vi "AVTCP-Test Client.vi"() -> ()   [LabVIEW 2016]
panel:
  out "result":i32
  in  "Send":bool
  in  "stop":bool
  in  "Message":string
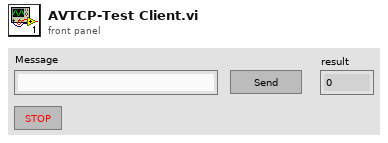
[diagram p1: front panel]
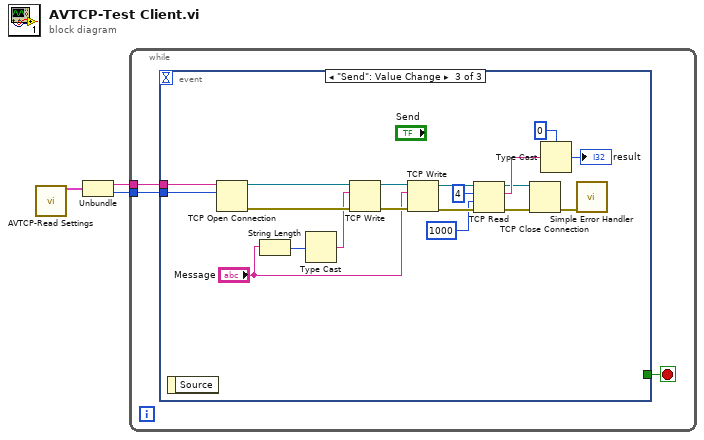
[diagram p0: block diagram]
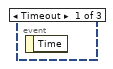
[diagram p2: hidden frame]
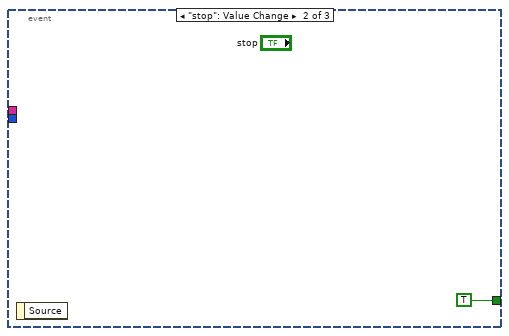
[diagram p3: hidden frame]
diagram:
  n1 = call "AVTCP-Read Settings.vi"() -> ("TCP"=w3:cluster{"IP Address":string, "Port":i32})  [unwired: 14 in, 1 out]
  n2 = Unbundle(w3) -> ("IP Address"=w2:string, "Port"=w1:i32)
  n3 = while {
    tunnel: w2 -> [w5]
    tunnel: w1 -> [w4]
    stop <- w6 stop-if-true
    n4 = event shown="[2] \"Send\": Value Change" {
      selector: _ -> [_ _ _]
      dyn-events: _ -> [_ _ _]
      timeout: _ -> [_ _ _]
      tunnel: [_ TRUE _] -> w6
      tunnel: w5 -> [_ _ w26]
      tunnel: w4 -> [_ _ w25]
      event Timeout {
        n5 = event-data() -> ()  [unwired: 1 in, 1 out]
      }
      event "stop": Value Change {
        n6 = event-data() -> ()  [unwired: 1 in, 1 out]
      }
      event "Send": Value Change {
        n7 = event-data() -> ()  [unwired: 1 in, 1 out]
        n8 = TCP Open Connection(address=w26, remote port or service name=w25) -> (connection ID=w14:refnum<k5>, error out=w11:errorcluster)  [unwired: 3 in]
        n9 = String Length(string="Message") -> (length=w9:i32)
        n10 = Type Cast(x=w9) -> (*(type *) &x=w8:string)  [unwired: 1 in]
        n11 = TCP Write(connection ID=w14, data in=w8, error in (no error)=w11) -> (connection ID out=w13:refnum<k5>, error out=w12:errorcluster)  [unwired: 1 in, 1 out]
        n12 = TCP Write(connection ID=w13, data in="Message", error in (no error)=w12) -> (connection ID out=w23:refnum<k5>, error out=w24:errorcluster)  [unwired: 1 in, 1 out]
        n13 = TCP Read(connection ID=w23, bytes to read=4, error in (no error)=w24, 9:1000 ("timeout ms (25000)")) -> (connection ID out=w17:refnum<k5>, data out=w21:string, error out=w18:errorcluster)  [unwired: 1 in]
        n14 = TCP Close Connection(connection ID=w17, error in (no error)=w18) -> (error out=w16:errorcluster)  [unwired: 1 in, 1 out]
        n15 = Type Cast(type=0, x=w21) -> (*(type *) &x=→"result":i32)
        n16 = call <vilib>:"Simple Error Handler.vi"("error in (no error)"=w16) -> ()  [unwired: 4 in, 5 out]
      }
    }
  }
